vi "Classify Error.vi"(8 "error in (no error)":errorcluster, 9 "Command Type (0)":i32, 10 "Message String":string, 11 "VISA resource name":refnum<visa-resource-name>) -> (0 "error out":errorcluster, 3 "VISA resource name out":refnum<visa-resource-name>)   [LabVIEW 2018, in "LTB-1.lvlib" / "3150.lvlib"]
doc: "Performs classification of error based on the mode of communication and the type of command. Identifies common messages from the instrument. Responsible for creating proper error message and logging into the error cluster."
uses:
  3150.lvlib
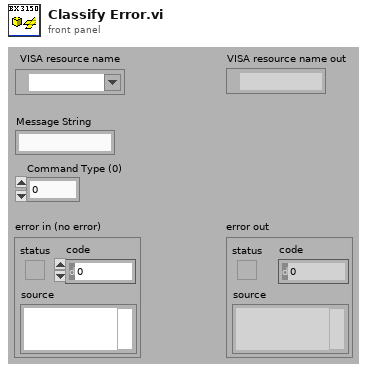
[diagram p1: front panel]
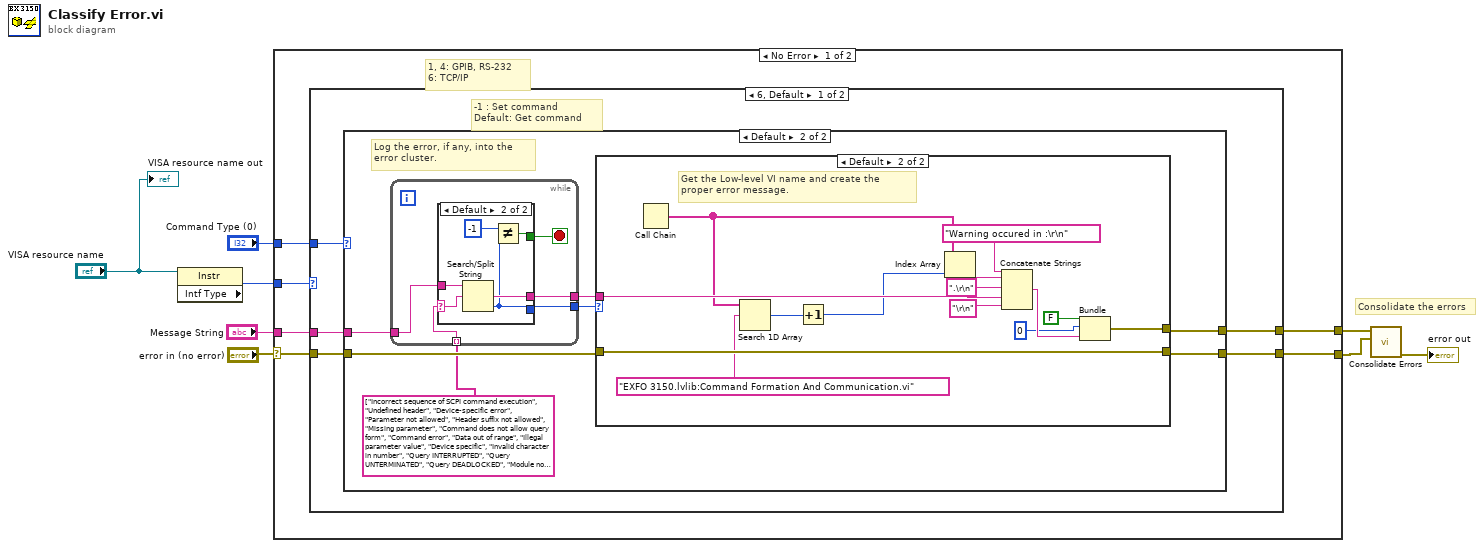
[diagram p0: block diagram]
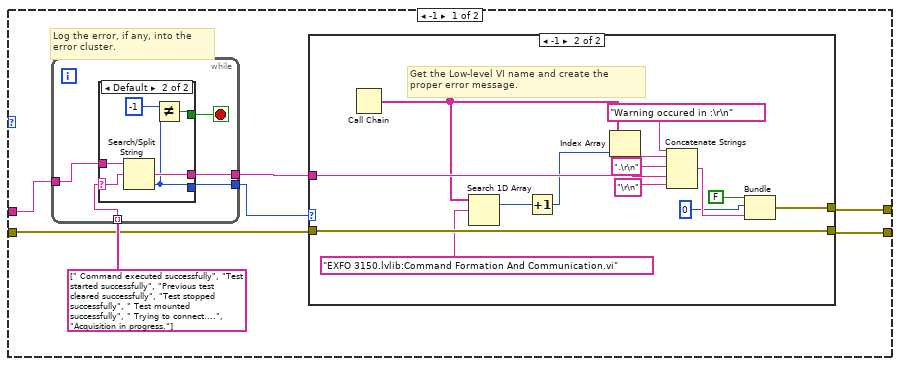
[diagram p2: hidden frame]
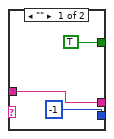
[diagram p3: hidden frame]
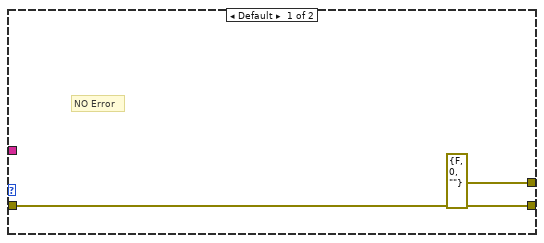
[diagram p4: hidden frame]
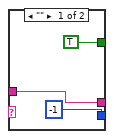
[diagram p5: hidden frame]
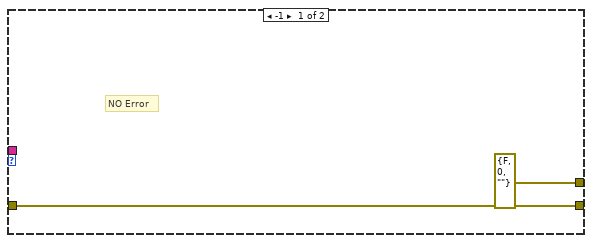
[diagram p6: hidden frame]
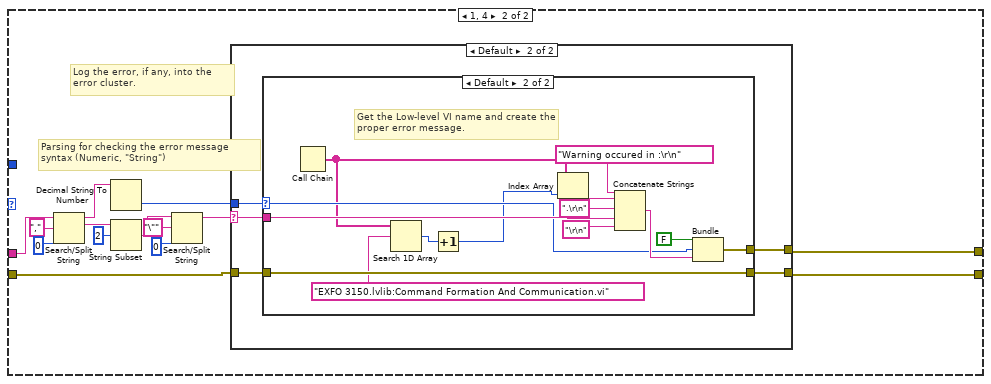
[diagram p7: hidden frame]
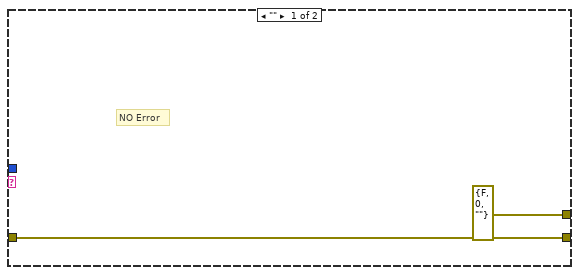
[diagram p8: hidden frame]
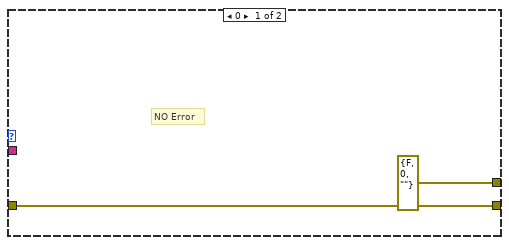
[diagram p9: hidden frame]
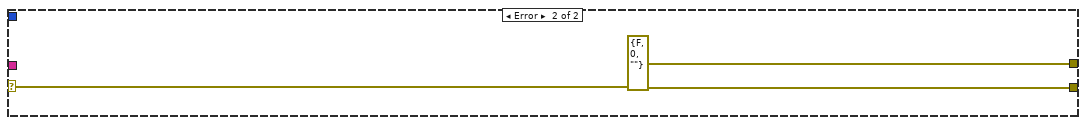
[diagram p10: hidden frame]
diagram:
  # "Consolidate the errors"
  n1 = property class="Instr"(reference="VISA resource name") -> ("Intf Type"=w7:u16)  [unwired: 1 in, 2 out]
  n2 = case shown="No Error" "error in (no error)" {
    selector: "error in (no error)" -> [w12 w132]
    tunnel: [w13 w132] -> w3
    tunnel: "Message String" -> [w14 _]
    tunnel: [w11 errorcluster {"status"=FALSE, "code"=0, "source"=""} ("error IO")] -> w4
    tunnel: w7 -> [w10 _]
    tunnel: "Command Type (0)" -> [w9 _]
    frame No Error {
      # "1, 4: GPIB, RS-232\n6: TCP/IP"
      # "ErrorMng"
      n3 = case shown="6, Default" w10 {
        tunnel: w14 -> [w16 w103]
        tunnel: [w18 w98] -> w13
        tunnel: w12 -> [w17 w97]
        tunnel: [w19 w94] -> w11
        tunnel: w9 -> [w15 _]
        frame 6, Default {
          # "-1 : Set command\nDefault: Get command"
          n4 = case shown="Default" w15 {
            tunnel: [w26 w63] -> w19
            tunnel: [w25 w62] -> w18
            tunnel: w17 -> [w20 w61]
            tunnel: w16 -> [w23 w60]
            frame -1 {
              # "Log the error, if any, into the\nerror cluster."
              n5 = while {
                tunnel: w23 -> [w31]
                tunnel: [w30] -> w21
                tunnel: [w29] -> w22
                tunnel: string[] [" Command executed successfully", "Test started successfully", "Previous test cleared successfully", "Test stopped successfully", " Test mounted successfully", " Trying to connect....", "Acquisition in progress."] -> [w28] mode=indexing
                stop <- w27 stop-if-true
                n6 = case shown="Default" w28 {
                  selector: w28 -> [_ w38]
                  tunnel: w31 -> [w34 w40]
                  tunnel: [-1 ("offset of match") w36] -> w30
                  tunnel: [w34 w39] -> w29
                  tunnel: [TRUE w37] -> w27
                  frame "" {
                  }
                  frame Default {
                    n7 = Search/Split String(string=w40, search string/char (-)=w38) -> (match + rest of string=w39:string, offset of match=w36:i32)  [unwired: 2 out]
                    n8 = Not Equal?(x=-1, y=w36) -> (x != y?=w37:bool)
                  }
                }
              }
              n9 = case shown="-1" w21 {
                tunnel: [w42 w56] -> w25
                tunnel: w20 -> [w42 w56]
                tunnel: [errorcluster {"status"=FALSE, "code"=0, "source"=""} ("error IO") w55] -> w26
                tunnel: w22 -> [_ w48]
                frame Default {
                  # "NO Error"
                }
                frame -1 {
                  # "Get the Low-level VI name and create the\nproper error message."
                  n10 = Call Chain() -> (call chain=w46:string[])
                  n11 = Search 1D Array(1D array=w46, element="EXFO 3150.lvlib:Command Formation And Communication.vi") -> (index of element=w44:i32)  [unwired: 1 out]
                  n12 = Increment(x=w44) -> (x+1=w43:i32)
                  n13 = Index Array(array=w46, index=w43) -> (element=w52:string)
                  n14 = Concatenate Strings("Warning occured in :\r\n", w52, ".\r\n", w48, "\r\n") -> (w49:string)
                  n15 = Bundle(FALSE, "number"=0, w49) -> (w55:cluster{bool, "number":i32, string})  [unwired: 1 out]
                }
              }
            }
            frame Default {
              # "Log the error, if any, into the\nerror cluster."
              n16 = while {
                tunnel: w60 -> [w68]
                tunnel: [w67] -> w59
                tunnel: [w66] -> w58
                tunnel: string[] ["Incorrect sequence of SCPI command execution", "Undefined header", "Device-specific error", "Parameter not allowed", "Header suffix not allowed", "Missing parameter", "Command does not allow query form", "Command error", "Data out of range", "Illegal parameter value", "Device specific", "Invalid character in number", "Query INTERRUPTED", "Query UNTERMINATED", "Query DEADLOCKED", "Module not present on slot", "Unable to retrieve data", "The command not support the query form", "Power control option not available."] -> [w65] mode=indexing
                stop <- w64 stop-if-true
                n17 = case shown="Default" w65 {
                  selector: w65 -> [_ w75]
                  tunnel: w68 -> [w71 w77]
                  tunnel: [-1 ("offset of match") w73] -> w67
                  tunnel: [w71 w76] -> w66
                  tunnel: [TRUE w74] -> w64
                  frame "" {
                  }
                  frame Default {
                    n18 = Search/Split String(string=w77, search string/char (-)=w75) -> (match + rest of string=w76:string, offset of match=w73:i32)  [unwired: 2 out]
                    n19 = Not Equal?(x=-1, y=w73) -> (x != y?=w74:bool)
                  }
                }
              }
              n20 = case shown="Default" w59 {
                tunnel: [w79 w93] -> w62
                tunnel: w61 -> [w79 w93]
                tunnel: [errorcluster {"status"=FALSE, "code"=0, "source"=""} ("error IO") w92] -> w63
                tunnel: w58 -> [_ w85]
                frame -1 {
                  # "NO Error"
                }
                frame Default {
                  # "Get the Low-level VI name and create the\nproper error message."
                  n21 = Call Chain() -> (call chain=w83:string[])
                  n22 = Search 1D Array(1D array=w83, element="EXFO 3150.lvlib:Command Formation And Communication.vi") -> (index of element=w81:i32)  [unwired: 1 out]
                  n23 = Increment(x=w81) -> (x+1=w80:i32)
                  n24 = Index Array(array=w83, index=w80) -> (element=w89:string)
                  n25 = Concatenate Strings("Warning occured in :\r\n", w89, ".\r\n", w85, "\r\n") -> (w86:string)
                  n26 = Bundle(FALSE, "number"=0, w86) -> (w92:cluster{bool, "number":i32, string})  [unwired: 1 out]
                }
              }
            }
          }
        }
        frame 1, 4 {
          # "Parsing for checking the error message\nsyntax (Numeric, \"String\")"
          # "Log the error, if any, into the\nerror cluster."
          n27 = Search/Split String(string=w103, search string/char (-)=",", offset (0)=0) -> (substring before match=w104:string, match + rest of string=w100:string)  [unwired: 1 out]
          n28 = Decimal String To Number(string=w104) -> (number=w96:i32)  [unwired: 3 out]
          n29 = String Subset(string=w100, offset (0)=2) -> (substring=w99:string)  [unwired: 1 out]
          n30 = Search/Split String(string=w99, search string/char (-)="\"", offset (0)=0) -> (substring before match=w95:string)  [unwired: 2 out]
          n31 = case shown="Default" w95 {
            selector: w95 -> [_ w111]
            tunnel: [w109 w114] -> w98
            tunnel: w97 -> [w109 w113]
            tunnel: w96 -> [_ w112]
            tunnel: [errorcluster {"status"=FALSE, "code"=0, "source"=""} ("error IO") w110] -> w94
            frame "" {
              # "NO Error"
            }
            frame Default {
              n32 = case shown="Default" w112 {
                selector: w112 -> [_ w123]
                tunnel: w111 -> [_ w125]
                tunnel: [w116 w121] -> w114
                tunnel: w113 -> [w116 w121]
                tunnel: [errorcluster {"status"=FALSE, "code"=0, "source"=""} ("error IO") w122] -> w110
                frame 0 {
                  # "NO Error"
                }
                frame Default {
                  # "Get the Low-level VI name and create the\nproper error message."
                  n33 = Call Chain() -> (call chain=w120:string[])
                  n34 = Search 1D Array(1D array=w120, element="EXFO 3150.lvlib:Command Formation And Communication.vi") -> (index of element=w118:i32)  [unwired: 1 out]
                  n35 = Increment(x=w118) -> (x+1=w117:i32)
                  n36 = Index Array(array=w120, index=w117) -> (element=w128:string)
                  n37 = Concatenate Strings("Warning occured in :\r\n", w128, ".\r\n", w125, "\r\n") -> (w124:string)
                  n38 = Bundle(FALSE, w123, w124) -> (w122:errorcluster)  [unwired: 1 out]
                }
              }
            }
          }
        }
      }
    }
    frame Error {
    }
  }
  n39 = call "Consolidate Errors.vi"("error existing"=w3, "error new"=w4) -> ("error out"=→"error out":errorcluster)  [unwired: 9 out]
  "VISA resource name out" <- "VISA resource name"
